vi "ScaleBias2.vi"(4 "AmpIN":waveform(dbl), 6 "VacIN":waveform(dbl), 8 "ScaleBias 2":T1={"Scale"=100.0, "Bias"=100.0} {"Bias" format="%#_13g"; "Scale" format="%#_13g"}, 11 "ScaleBias":T1={"Scale"=100.0, "Bias"=100.0} {"Bias" format="%#_13g"; "Scale" format="%#_13g"}) -> (3 "Cluster":T2)   [LabVIEW 2013]
uses:
  ScaleBias.ctl
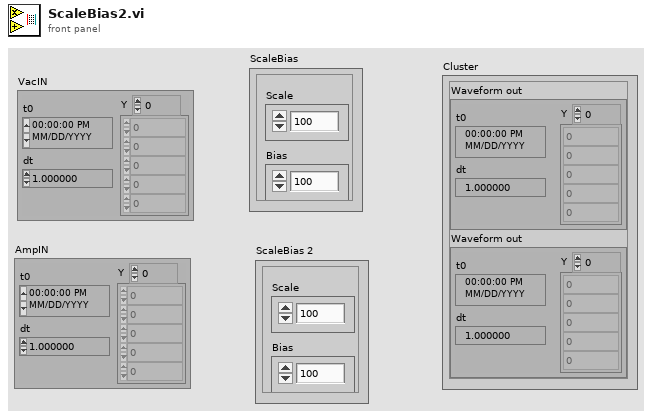
[diagram p1: front panel]
types:
  T1 = typedef "ScaleBias.ctl" = cluster{"Scale":dbl, "Bias":dbl}
  T2 = cluster{"Waveform out":waveform(dbl), "Waveform out":waveform(dbl)}
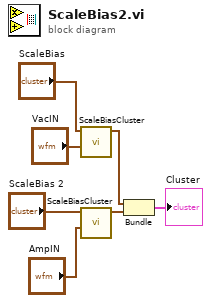
[diagram p0: block diagram]
diagram:
  n1 = call "ScaleBiasCluster.vi"("Waveform in"="VacIN", "ScaleBias"="ScaleBias") -> ("Waveform out"=w2:waveform(dbl))  [unwired: 9 in]
  n2 = call "ScaleBiasCluster.vi"("Waveform in"="AmpIN", "ScaleBias"="ScaleBias 2") -> ("Waveform out"=w5:waveform(dbl))  [unwired: 9 in]
  n3 = Bundle("Waveform out"=w2, "Waveform out"=w5) -> (→"Cluster":T2)  [unwired: 1 in]
